vi "Construct Terminal Enabled State Binding.vi"(7 "Initial State (T)":bool=TRUE, 8 "FALSE State (Disabled and Grayed Out)":T1(ring)=enum."Disabled and Grayed Out", 9 "TRUE State (Enabled)":T1(ring), 10 "Control":refnum<vi>) -> (0 "error out":errorcluster, 3 "TerminalEnabledStateBinding":refnum<class "TerminalEnabledStateBinding.lvclass">)   [LabVIEW 2019, in "TerminalEnabledStateBinding.lvclass"]
doc: "<License>\nCopyright © 2017 Composed Systems, LLC | All rights reserved\nwww.composed.io\n\nAuthor: Ethan Stern <ethan.stern@composed.io>\n\nThis software is provided \"AS IS\" WITHOUT WARRANTIES, either express or implied, AND IS FOR EDUCATIONAL PURPOSES ONLY.\n</License>"
uses:
  <vilib>/gpm_packages/@cs/transport/Source/Concrete/TerminalEnabledStateBinding/TerminalEnabledStateBinding.lvclass
  C:/Program Files/National Instruments/LabVIEW 2019/vi.lib/gpm_packages/@cs/transport/Source/Concrete/TerminalPropertyBinding/TerminalPropertyBinding.lvclass
  <vilib>/gpm_packages/@cs/transport/Source/Concrete/TerminalPropertyBinding/TerminalPropertyBinding.lvclass/TerminalPropertyBinding.ctl
  <vilib>/gpm_packages/@cs/transport/Source/Concrete/TerminalEnabledStateBinding/TerminalEnabledStateBinding.lvclass/TerminalEnabledStateBinding.ctl
  <vilib>/gpm_packages/@cs/transport/Source/Concrete/TerminalPropertyBinding/TerminalPropertyBinding.lvclass
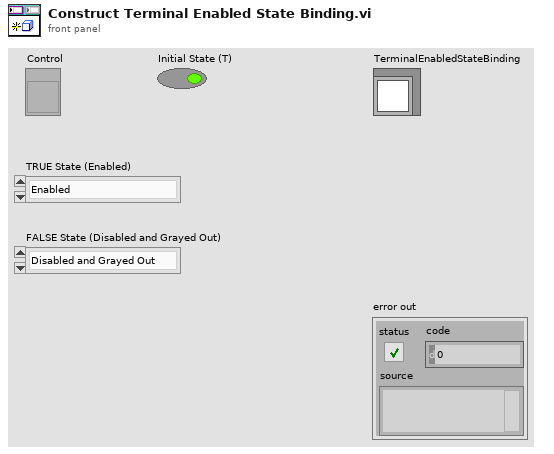
[diagram p1: front panel]
types:
  T1 = enum8{"Enabled", "Disabled", "Disabled and Grayed Out"}
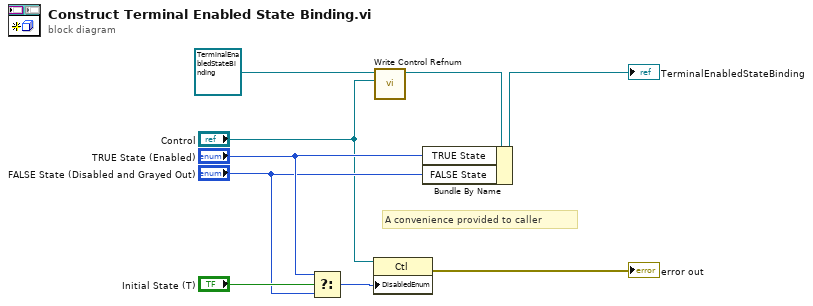
[diagram p0: block diagram]
diagram:
  # "A convenience provided to caller"
  n1 = Select(t="TRUE State (Enabled)", s="Initial State (T)", f="FALSE State (Disabled and Grayed Out)") -> (s? t:f=w4:T1)
  n2 = property class="Ctl"(reference="Control", "DisabledEnum"=w4) -> (error out=→"error out":errorcluster)  [unwired: 1 in, 1 out]
  n3 = call <vilib>:"Write Control Refnum.vi"("Ctl Refnum"="Control", "TerminalReference in"=refnum<class "TerminalEnabledStateBinding.lvclass"> refnum ("TerminalEnabledStateBinding.lvclass")) -> ("TerminalReferenceBinding Out"=w2:refnum<class "TerminalEnabledStateBinding.lvclass">)  [unwired: 9 in]
  n4 = Bundle By Name(cluster=w2, "TRUE State"="TRUE State (Enabled)", "FALSE State"="FALSE State (Disabled and Grayed Out)") -> (→"TerminalEnabledStateBinding":refnum<class "TerminalEnabledStateBinding.lvclass">)
